vi "Draw_star.vi"(8 "size":dbl, 10 "DEC (°)":dbl, 11 "RA (°)":dbl) -> (0 "Y":dbl[](array[numeric]) format="%.2g", 3 "X":dbl[](array[numeric]) format="%.2g")   [LabVIEW 2011]
panel:
  # "(0,5)"
  # "(2)"
  # "(3)"
  # "(4)"
  # "(1)"
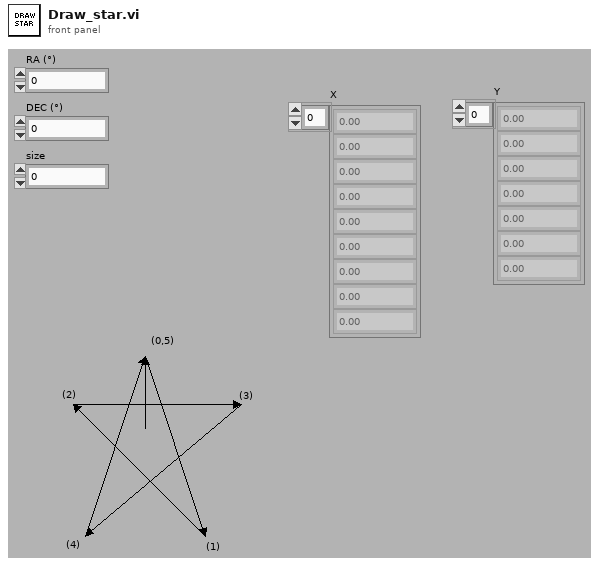
[diagram p1: front panel]
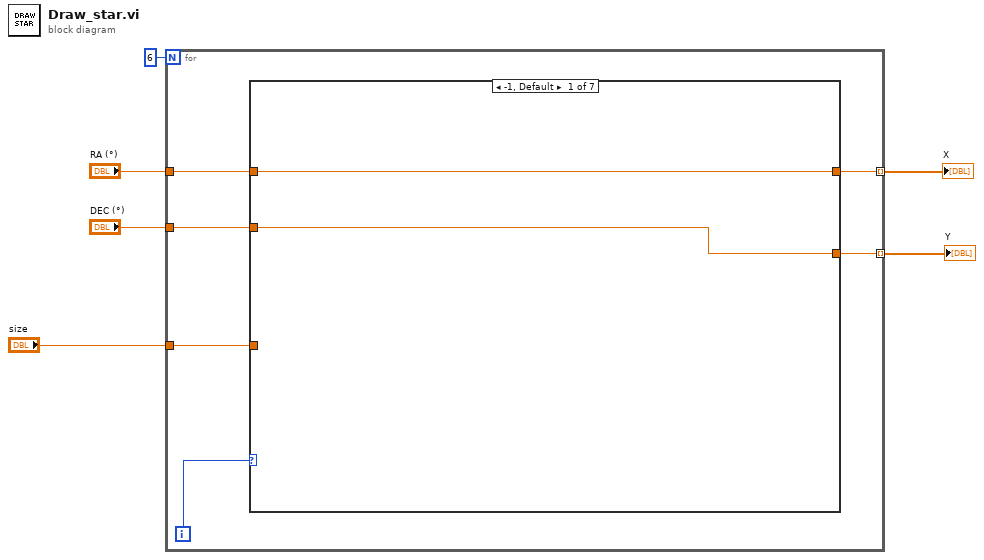
[diagram p0: block diagram]
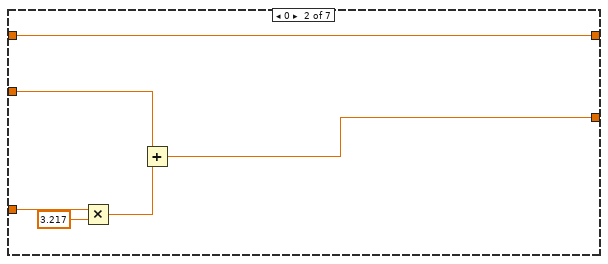
[diagram p2: hidden frame]
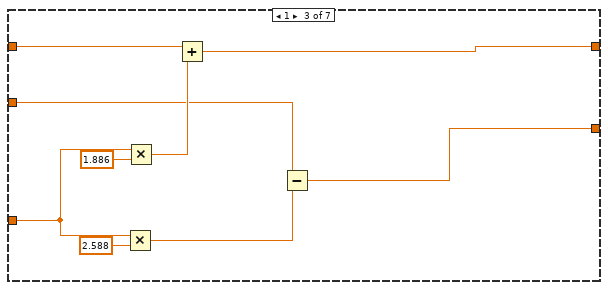
[diagram p3: hidden frame]
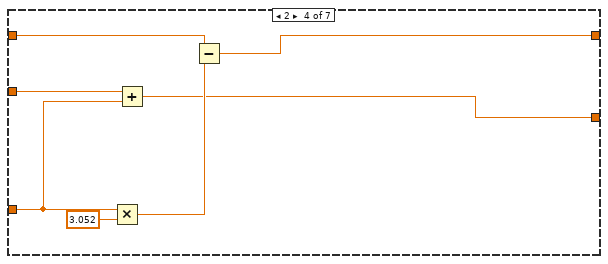
[diagram p4: hidden frame]
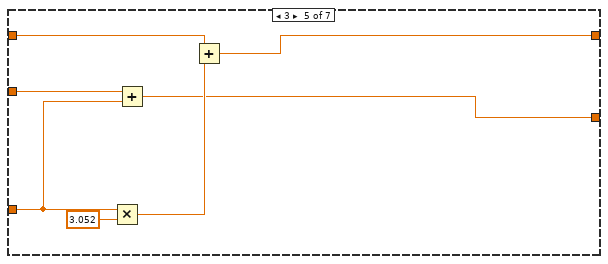
[diagram p5: hidden frame]
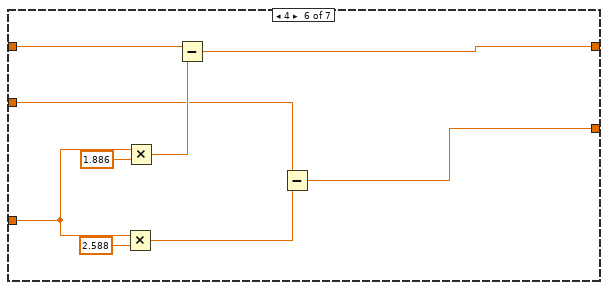
[diagram p6: hidden frame]
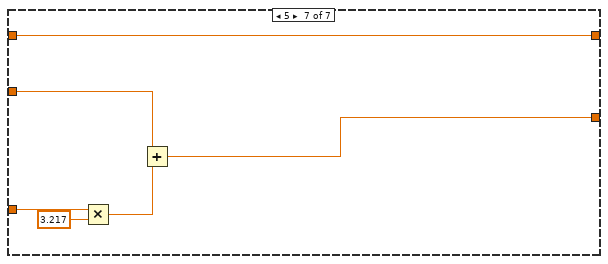
[diagram p7: hidden frame]
diagram:
  n1 = for {
    N: 6 -> [_]
    tunnel: [w8] -> w3 mode=indexing
    tunnel: [w7] -> w2 mode=indexing
    tunnel: "size" -> [w9]
    tunnel: "DEC (°)" -> [w10]
    tunnel: "RA (°)" -> [w11]
    i -> [w12]
    n2 = case shown="-1, Default" w12 {
      tunnel: w11 -> [w14 w19 w27 w36 w43 w50 w57]
      tunnel: w10 -> [w13 w20 w23 w33 w40 w46 w58]
      tunnel: w9 -> [_ w17 w29 w32 w39 w52 w55]
      tunnel: [w14 w19 w22 w30 w37 w45 w57] -> w8
      tunnel: [w13 w18 w21 w31 w38 w44 w56] -> w7
      frame -1, Default {
      }
      frame 0 {
        n3 = Multiply(x=w17, y=3.217) -> (x*y=w15:dbl)
        n4 = Add(x=w20, y=w15) -> (x+y=w18:dbl)
      }
      frame 1 {
        n5 = Multiply(x=w29, y=2.588) -> (x*y=w24:dbl)
        n6 = Multiply(x=w29, y=1.886) -> (x*y=w26:dbl)
        n7 = Add(x=w27, y=w26) -> (x+y=w22:dbl)
        n8 = Subtract(x=w23, y=w24) -> (x-y=w21:dbl)
      }
      frame 2 {
        n9 = Multiply(x=w32, y=3.052) -> (x*y=w34:dbl)
        n10 = Add(x=w33, y=w32) -> (x+y=w31:dbl)
        n11 = Subtract(x=w36, y=w34) -> (x-y=w30:dbl)
      }
      frame 3 {
        n12 = Multiply(x=w39, y=3.052) -> (x*y=w41:dbl)
        n13 = Add(x=w40, y=w39) -> (x+y=w38:dbl)
        n14 = Add(x=w43, y=w41) -> (x+y=w37:dbl)
      }
      frame 4 {
        n15 = Multiply(x=w52, y=2.588) -> (x*y=w47:dbl)
        n16 = Multiply(x=w52, y=1.886) -> (x*y=w49:dbl)
        n17 = Subtract(x=w50, y=w49) -> (x-y=w45:dbl)
        n18 = Subtract(x=w46, y=w47) -> (x-y=w44:dbl)
      }
      frame 5 {
        n19 = Multiply(x=w55, y=3.217) -> (x*y=w53:dbl)
        n20 = Add(x=w58, y=w53) -> (x+y=w56:dbl)
      }
    }
  }
  "X" <- w3
  "Y" <- w2
